vi "Oscilloscope.vi"() -> ()   [LabVIEW 2015]
uses:
  <vilib>/sound2/lvsound2.llb/Sampling Mode.ctl
  <vilib>/sound2/lvsound2.llb/Sound Data Format.ctl
  <vilib>/sound2/lvsound2.llb/Sound Input Read (DBL).vi
  <vilib>/Waveform/WDTOps.llb/WDT Index Channel DBL.vi
  <vilib>/measure/matone.llb/Extract Single Tone Information N Chan.vi
  <vilib>/express/express analysis/Spectral/Block/exnSpectralBlock spectral measurements power poly.vi
  <vilib>/express/express analysis/Spectral/Block/exnSpectralBlock spectral measurements power array WFM.vi
  <vilib>/express/express analysis/Spectral/XNode/ExpressSpectralMeasurementsBlockNode.xnode
  <vilib>/measure/NI_MAPro.lvlib
panel:
  in  "TRIGGER":enum32{"CHANNEL 1", "CHANNEL 2"}(radio)
  out "Amplitude (V)":dbl
  out "Amplitude (V)":dbl
  out "Frequency (Hz)":dbl
  out "Frequency (Hz)":dbl
  in  "Frequency Span [Hz]":dbl(knob) scale=1.0..50000.0
  in  "Channel 2":bool
  in  "Channel 1":bool
  in  "Amplitude [V]":dbl(knob) scale=0.001..1.0
  in  "Time [s]":dbl(knob) scale=1e-05..0.1
  in  "?":bool
  in  "?":T1(tab)
  out "Oscilloscope":dynamicdata(graph)
  out "Oscilloscope 2":cluster{"f0":dbl, "df":dbl, "magnitude":dbl[]}[](graph)
  out "Oscilloscope 3":cluster{"Y":dbl[], "Y":dbl[]}(graph)
  # "CHANNEL 1"
  # "CHANNEL 2"
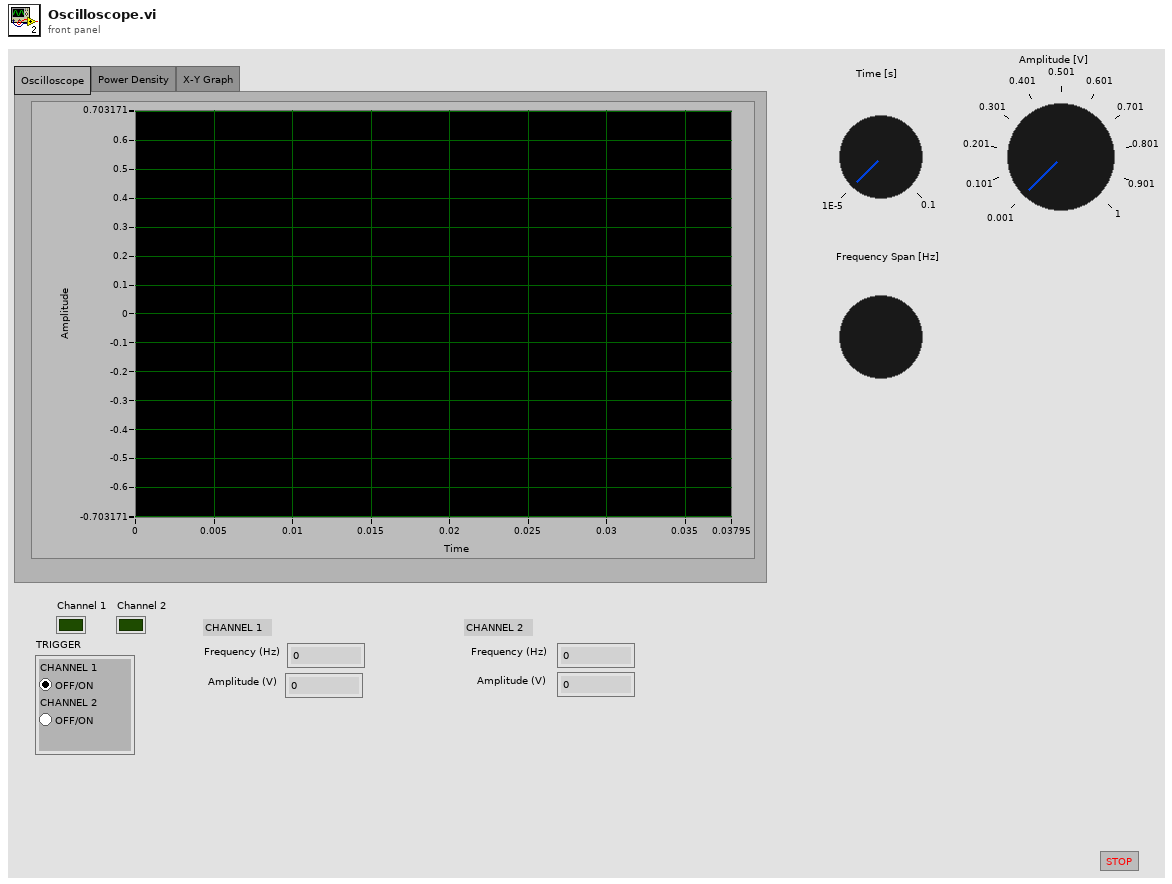
[diagram p1: front panel]
types:
  T1 = enum32{"Oscilloscope", "Power Density", "X-Y Graph"}
  T2 = typedef "Sound Data Format.ctl" = cluster{"sample rate (S/s)":dbl, "number of channels":i32, "bits per sample":i32}
  T3 = typedef "Sampling Mode.ctl" = i32
  T4 = typedef "Sound Input Task ID.ctl" = u32
  T5 = cluster{"averaging mode":u16, "weighting mode":u16, "number of averages":u32}
  T6 = cluster{"dB On (F)":bool, "unwrap phase (F)":bool, "convert to degree (F)":bool}
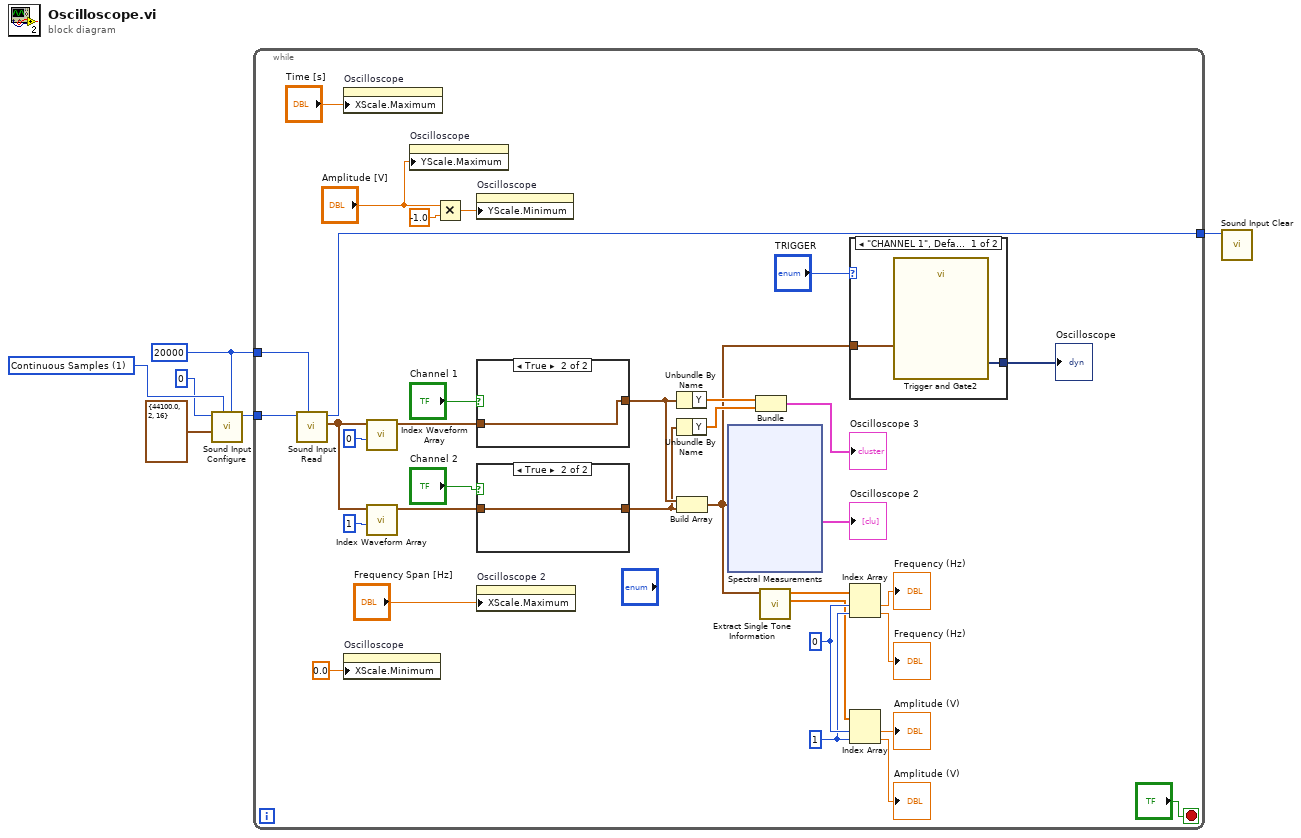
[diagram p0: block diagram]
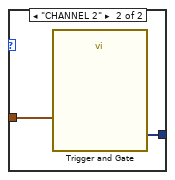
[diagram p2: hidden frame]
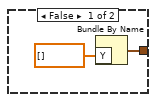
[diagram p3: hidden frame]
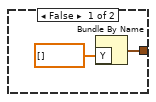
[diagram p4: hidden frame]
diagram:
  w2 = 20000
  w6 = T3 1 items=["Finite Samples", "Continuous Samples"] ("sample mode")
  n1 = call <vilib>:"Sound Input Configure.vi"("number of samples/ch"=w2, "sample mode"=w6, "sound format"=T2 {"sample rate (S/s)"=44100.0, "number of channels"=2, "bits per sample"=16} ("Sound Format"), "device ID"=0) -> ("task ID"=w4:T4)  [unwired: 6 in, 1 out]
  n2 = while {
    tunnel: w4 -> [w38]
    tunnel: w2 -> [w39]
    tunnel: [w37] -> w3
    stop <- "?" stop-if-true
    w19 = 1
    w20 = 0
    n3 = call-poly <vilib>:"Sound Input Read.vi"("number of samples/ch"=w39, "task ID"=w38) -> ("data"=w32:waveform(dbl)[], "task ID out"=w37:T4)  [unwired: 7 in, 1 out]
    n4 = property on="Oscilloscope" class="WFGraph (strict)"("XScale.Maximum"="Time [s]") -> ()  [unwired: 2 in, 2 out]
    n5 = property on="Oscilloscope" class="WFGraph (strict)"("XScale.Minimum"=0.0 ("X Scale.Range:Minimum")) -> ()  [unwired: 2 in, 2 out]
    n6 = call-poly <vilib>:"Index Waveform Array.vi"("index"=0, "waveform array"=w32) -> ("waveform"=w10:waveform(dbl))  [unwired: 8 in, 1 out]
    n7 = call-poly <vilib>:"Index Waveform Array.vi"("index"=1, "waveform array"=w32) -> ("waveform"=w11:waveform(dbl))  [unwired: 8 in, 1 out]
    n8 = property on="Oscilloscope" class="WFGraph (strict)"("YScale.Maximum"="Amplitude [V]") -> ()  [unwired: 2 in, 2 out]
    n9 = Multiply(x="Amplitude [V]", y=-1.0 ("x*y")) -> (x*y=w29:dbl)
    n10 = property on="Oscilloscope" class="WFGraph (strict)"("YScale.Minimum"=w29) -> ()  [unwired: 2 in, 2 out]
    n11 = case shown="True" "Channel 1" {
      tunnel: w10 -> [_ w59]
      tunnel: [w58 w59] -> w17
      frame False {
        n12 = Bundle By Name("Y"=dbl[] []) -> (w58:waveform(dbl))  [unwired: 1 in]
      }
      frame True {
      }
    }
    n13 = case shown="True" "Channel 2" {
      tunnel: w11 -> [_ w56]
      tunnel: [w55 w56] -> w16
      frame False {
        n14 = Bundle By Name("Y"=dbl[] []) -> (w55:waveform(dbl))  [unwired: 1 in]
      }
      frame True {
      }
    }
    n15 = property on="Oscilloscope 2" class="WFGraph (strict)"("XScale.Maximum"="Frequency Span [Hz]") -> ()  [unwired: 2 in, 2 out]
    n16 = Unbundle By Name(w17) -> ("Y"=w14:dbl[])
    n17 = Unbundle By Name(w16) -> ("Y"=w13:dbl[])
    n18 = Build Array(w17, w16) -> (w7:waveform(dbl)[])
    n19 = xnode "Spectral Measurements"("Signals"=w7) -> ("Power Spectrum"=→"Oscilloscope 2":cluster{"f0":dbl, "df":dbl, "magnitude":dbl[]}[])  [unwired: 1 in, 1 out]
    n20 = Bundle("Y"=w14, "Y"=w13) -> (→"Oscilloscope 3":cluster{"Y":dbl[], "Y":dbl[]})  [unwired: 1 in]
    n21 = call-poly <vilib>:"Extract Single Tone Information.vi"("time signals in"=w7) -> ("detected amplitudes"=w18:dbl[], "detected frequencies"=w24:dbl[])  [unwired: 5 in, 4 out]
    n22 = case shown="\"CHANNEL 1\", Default" "TRIGGER" {
      tunnel: [w41 w44] -> w8
      tunnel: w7 -> [w42 w43]
      frame "CHANNEL 1", Default {
        n23 = call "Trigger and Gate2"("Signals"=w42) -> ("Triggered Signals"=w41:dynamicdata)  [unwired: 7 in, 3 out]
      }
      frame "CHANNEL 2" {
        n24 = call "Trigger and Gate"("Signals"=w43) -> ("Triggered Signals"=w44:dynamicdata)  [unwired: 7 in, 3 out]
      }
    }
    "Oscilloscope" <- w8
    n25 = Index Array(array=w24, index #1=w20, index #2=w19) -> (element #1=→"Frequency (Hz)":dbl, element #2=→"Frequency (Hz)":dbl)
    n26 = Index Array(array=w18, index #1=w20, index #2=w19) -> (element #1=→"Amplitude (V)":dbl, element #2=→"Amplitude (V)":dbl)
  }
  n27 = call <vilib>:"Sound Input Clear.vi"("task ID"=w3) -> ()  [unwired: 10 in, 1 out]
